vi "Agilent VNA Set IFBW.vi"(6 "Channel":i8=1 min=1 max=99 step=1, 7 "Agilent VNA":T1, 8 "error in (no error)":errorcluster, 10 "IFBW, Hz (3000)":dbl=3000.0, 11 "VISA Resource Name":refnum<visa-resource-name>) -> (0 "error out":errorcluster, 3 "dup VISA Resource Name":refnum<visa-resource-name>)   [LabVIEW 2011]
doc: "This Vi for the HP8753B Network Analyzer is used to set averaging, smoothing, and the IF bandwidth."
uses:
  TypeDefs/Agilent VNA Instrument Info.ctl
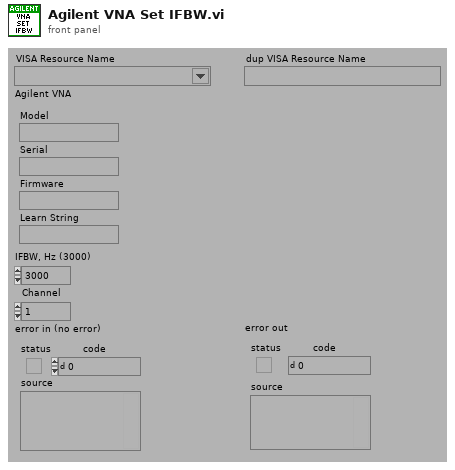
[diagram p1: front panel]
types:
  T1 = typedef "Agilent VNA Instrument Info.ctl" = cluster{"Model":string, "Serial":string, "Firmware":string, "Learn String":string}
  T2 = typedef "Agilent VNA Model.ctl" = enum16{"Not Supported", "8510X", "8719X", "8720X", "8722X", "8753X", "ENA", "PNA", "Field Fox"}
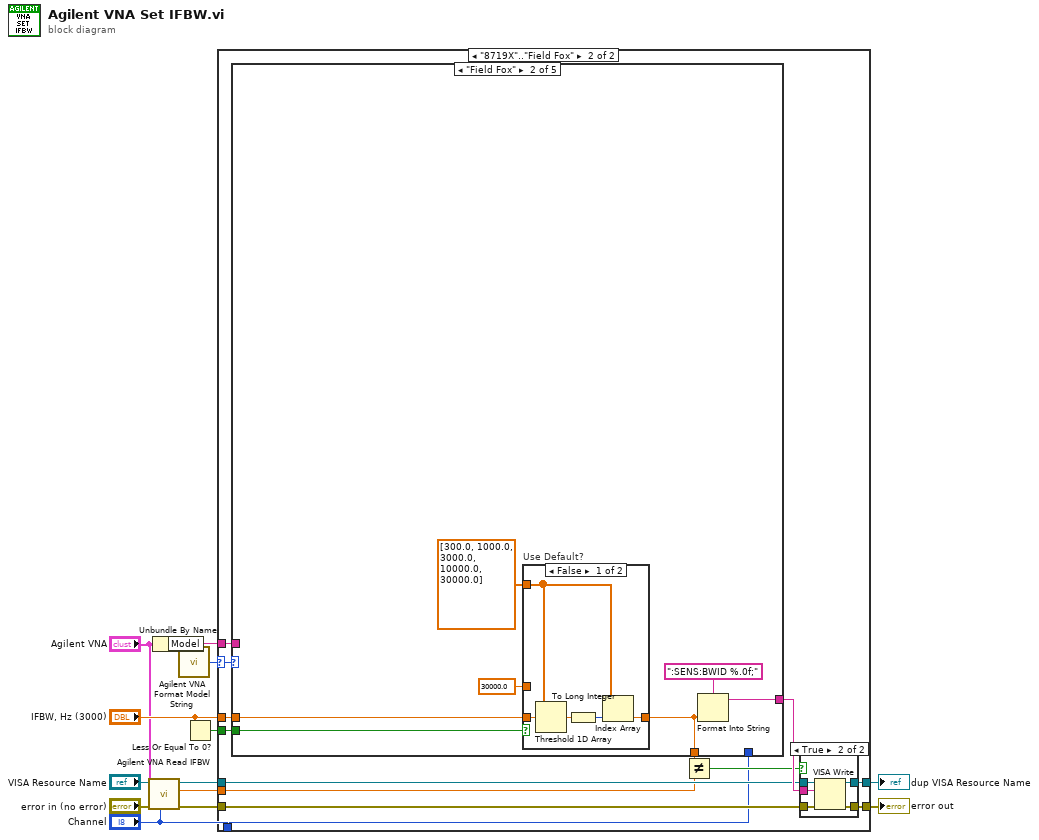
[diagram p0: block diagram]
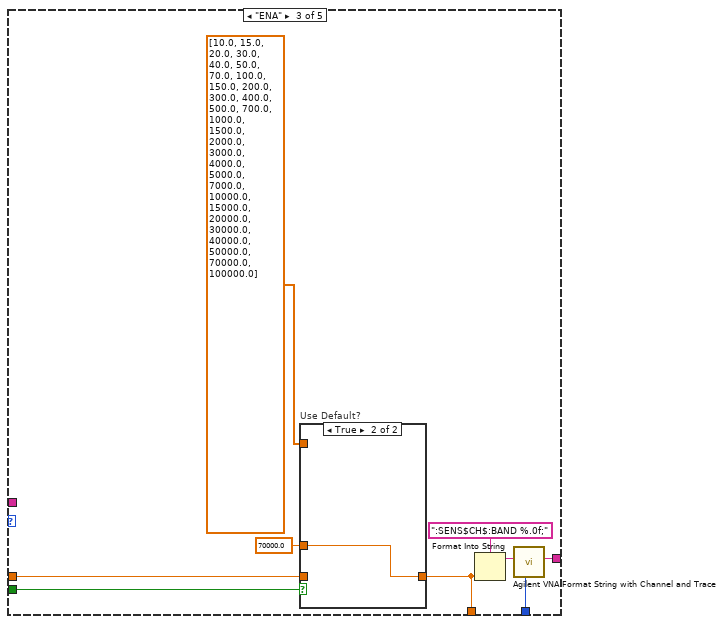
[diagram p5: hidden frame]
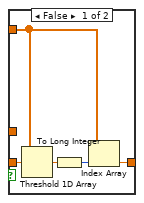
[diagram p6: hidden frame]
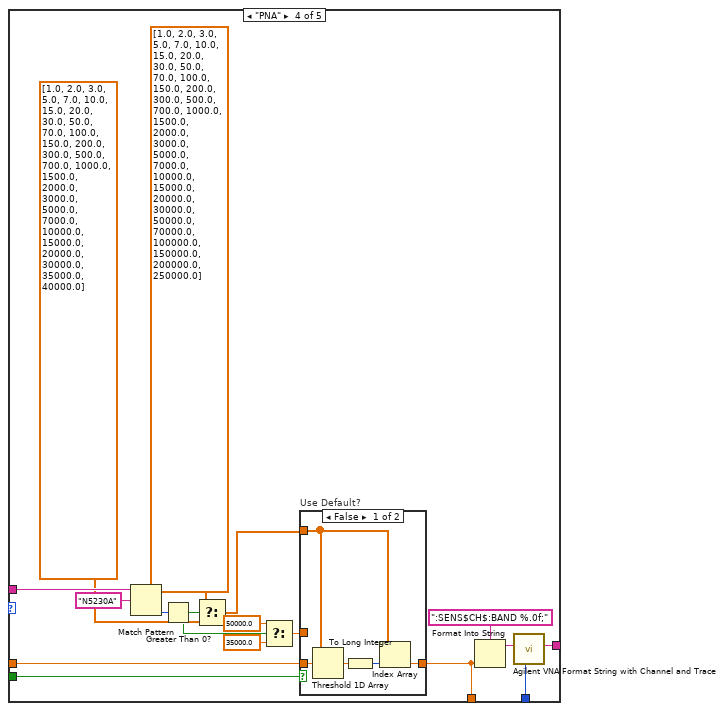
[diagram p7: hidden frame]
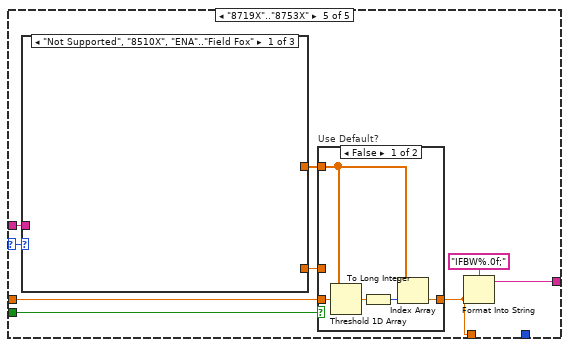
[diagram p9: hidden frame]
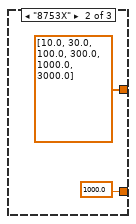
[diagram p11: hidden frame]
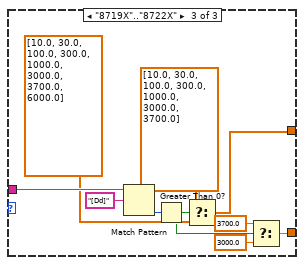
[diagram p12: hidden frame]
diagram:
  n1 = call "Agilent VNA Read IFBW.vi"("Channel"="Channel", "Agilent VNA"="Agilent VNA", "error in (no error)"="error in (no error)", "VISA Resource Name"="VISA Resource Name") -> ("error out"=w8:errorcluster, "IFBW, Hz"=w7:dbl, "dup VISA Resource Name"=w9:refnum<visa-resource-name>)  [unwired: 5 out]
  n2 = Unbundle By Name("Agilent VNA") -> ("Model"=w1:string)
  n3 = call "Agilent VNA Format Model String.vi"("Model"=w1) -> ("Model"=w3:T2)
  n4 = Less Or Equal To 0?(x="IFBW, Hz (3000)") -> (x <= 0?=w5:bool)
  n5 = case shown="\"8719X\"..\"Field Fox\"" w3 {
    selector: w3 -> [_ w18]
    tunnel: [w15 w28] -> w13
    tunnel: [w14 w27] -> w12
    tunnel: w9 -> [w14 w25]
    tunnel: w8 -> [w15 w24]
    tunnel: w7 -> [_ w22]
    tunnel: "IFBW, Hz (3000)" -> [_ w20]
    tunnel: w5 -> [_ w19]
    tunnel: "Channel" -> [_ w17]
    tunnel: w1 -> [_ w16]
    frame "Not Supported", "8510X" {
      # "The HP 8510 does not have the ability to set the IFBW."
    }
    frame "8719X".."Field Fox" {
      n6 = case shown="\"Field Fox\"" w18 {
        selector: w18 -> [_ _ _ _ w82]
        tunnel: w20 -> [_ w31 w46 w71 w87]
        tunnel: [_ w29 w43 w68 w85] -> w26
        tunnel: [_ w30 w45 w70 w83] -> w21
        tunnel: w19 -> [_ w34 w49 w72 w81]
        tunnel: w17 -> [_ _ w42 w67 _]
        tunnel: w16 -> [_ _ _ w65 w80]
        frame "Not Supported", "8510X" {
        }
        frame "Field Fox" {
          n7 = case "Use Default?" shown="False" w34 {
            tunnel: dbl[] [300.0, 1000.0, 3000.0, 10000.0, 30000.0] -> [w39 _]
            tunnel: w31 -> [w37 _]
            tunnel: [w36 w41] -> w30
            tunnel: 30000.0 -> [_ w41]
            frame False {
              n8 = Threshold 1D Array(2:w37, 3:w39) -> (0:w40:dbl)  [unwired: 1 out]
              n9 = To Long Integer(number=w40) -> (32bit integer=w38:i32)
              n10 = Index Array(array=w39, index=w38) -> (element=w36:dbl)
            }
            frame True {
            }
          }
          n11 = Format Into String(format string=":SENS:BWID %.0f;", w30) -> (resulting string=w29:string)  [unwired: 2 in, 1 out]
        }
        frame "ENA" {
          n12 = case "Use Default?" shown="True" w49 {
            tunnel: dbl[] [10.0, 15.0, 20.0, 30.0, 40.0, 50.0, 70.0, 100.0, 150.0, 200.0, 300.0, 400.0, 500.0, 700.0, 1000.0, 1500.0, 2000.0, 3000.0, 4000.0, 5000.0, 7000.0, 10000.0, 15000.0, 20000.0, 30000.0, 40000.0, 50000.0, 70000.0, 100000.0] -> [w54 _]
            tunnel: w46 -> [w52 _]
            tunnel: [w51 w56] -> w45
            tunnel: 70000.0 -> [_ w56]
            frame False {
              n13 = Threshold 1D Array(2:w52, 3:w54) -> (0:w55:dbl)  [unwired: 1 out]
              n14 = To Long Integer(number=w55) -> (32bit integer=w53:i32)
              n15 = Index Array(array=w54, index=w53) -> (element=w51:dbl)
            }
            frame True {
            }
          }
          n16 = Format Into String(format string=":SENS$CH$:BAND %.0f;", w45) -> (resulting string=w44:string)  [unwired: 2 in, 1 out]
          n17 = call "Agilent VNA Format String with Channel and Trace.vi"("Channel"=w42, "String"=w44) -> ("String Out"=w43:string)  [unwired: 1 in, 6 out]
        }
        frame "PNA" {
          n18 = Match Pattern(string=w65, regular expression="N5230A") -> (offset past match=w66:i32)  [unwired: 4 out]
          n19 = Greater Than 0?(x=w66) -> (x > 0?=w57:bool)
          n20 = Select(t=dbl[] [1.0, 2.0, 3.0, 5.0, 7.0, 10.0, 15.0, 20.0, 30.0, 50.0, 70.0, 100.0, 150.0, 200.0, 300.0, 500.0, 700.0, 1000.0, 1500.0, 2000.0, 3000.0, 5000.0, 7000.0, 10000.0, 15000.0, 20000.0, 30000.0, 50000.0, 70000.0, 100000.0, 150000.0, 200000.0, 250000.0], s=w57, f=dbl[] [1.0, 2.0, 3.0, 5.0, 7.0, 10.0, 15.0, 20.0, 30.0, 50.0, 70.0, 100.0, 150.0, 200.0, 300.0, 500.0, 700.0, 1000.0, 1500.0, 2000.0, 3000.0, 5000.0, 7000.0, 10000.0, 15000.0, 20000.0, 30000.0, 35000.0, 40000.0]) -> (s? t:f=w61:dbl[])
          n21 = Select(t=50000.0, s=w57, f=35000.0) -> (s? t:f=w59:dbl)
          n22 = case "Use Default?" shown="False" w72 {
            tunnel: w61 -> [w77 _]
            tunnel: w71 -> [w75 _]
            tunnel: [w74 w79] -> w70
            tunnel: w59 -> [_ w79]
            frame False {
              n23 = Threshold 1D Array(2:w75, 3:w77) -> (0:w78:dbl)  [unwired: 1 out]
              n24 = To Long Integer(number=w78) -> (32bit integer=w76:i32)
              n25 = Index Array(array=w77, index=w76) -> (element=w74:dbl)
            }
            frame True {
            }
          }
          n26 = Format Into String(format string=":SENS$CH$:BAND %.0f;", w70) -> (resulting string=w69:string)  [unwired: 2 in, 1 out]
          n27 = call "Agilent VNA Format String with Channel and Trace.vi"("Channel"=w67, "String"=w69) -> ("String Out"=w68:string)  [unwired: 1 in, 6 out]
        }
        frame "8719X".."8753X" {
          n28 = case shown="\"Not Supported\", \"8510X\", \"ENA\"..\"Field Fox\"" w82 {
            tunnel: [_ dbl[] [10.0, 30.0, 100.0, 300.0, 1000.0, 3000.0] w102] -> w88
            tunnel: [_ 1000.0 w98] -> w84
            tunnel: w80 -> [_ _ w105]
            frame "Not Supported", "8510X", "ENA".."Field Fox" {
            }
            frame "8753X" {
            }
            frame "8719X".."8722X" {
              n29 = Match Pattern(string=w105, regular expression="[Dd]") -> (offset past match=w104:i32)  [unwired: 4 out]
              n30 = Greater Than 0?(x=w104) -> (x > 0?=w97:bool)
              n31 = Select(t=dbl[] [10.0, 30.0, 100.0, 300.0, 1000.0, 3000.0, 3700.0], s=w97, f=dbl[] [10.0, 30.0, 100.0, 300.0, 1000.0, 3000.0, 3700.0, 6000.0]) -> (s? t:f=w102:dbl[])
              n32 = Select(t=3700.0, s=w97, f=3000.0) -> (s? t:f=w98:dbl)
            }
          }
          n33 = case "Use Default?" shown="False" w81 {
            tunnel: w88 -> [w92 _]
            tunnel: w87 -> [w90 _]
            tunnel: [w89 w94] -> w83
            tunnel: w84 -> [_ w94]
            frame False {
              n34 = Threshold 1D Array(2:w90, 3:w92) -> (0:w93:dbl)  [unwired: 1 out]
              n35 = To Long Integer(number=w93) -> (32bit integer=w91:i32)
              n36 = Index Array(array=w92, index=w91) -> (element=w89:dbl)
            }
            frame True {
            }
          }
          n37 = Format Into String(format string="IFBW%.0f;", w83) -> (resulting string=w85:string)  [unwired: 2 in, 1 out]
        }
      }
      n38 = Not Equal?(x=w21, y=w22) -> (x != y?=w23:bool)
      n39 = case shown="True" w23 {
        tunnel: [w107 w113] -> w28
        tunnel: [w108 w112] -> w27
        tunnel: w26 -> [_ w111]
        tunnel: w25 -> [w108 w110]
        tunnel: w24 -> [w107 w109]
        frame False {
        }
        frame True {
          n40 = VISA Write(VISA resource name=w110, write buffer=w111, error in (no error)=w109) -> (VISA resource name out=w112:refnum<visa-resource-name>, error out=w113:errorcluster)  [unwired: 1 out]
        }
      }
    }
  }
  "error out" <- w13
  "dup VISA Resource Name" <- w12
